vi "Draw Robot.vi"(7 "Gyro":dbl, 10 "XY":cluster{"X":dbl, "Y":dbl}) -> (2 "Graph 2":cluster{cluster{"X":dbl, "Y":dbl}[]}[](graph))   [LabVIEW 2018]
panel:
  in  "Robot Lenght":dbl
  in  "Robot Width":dbl
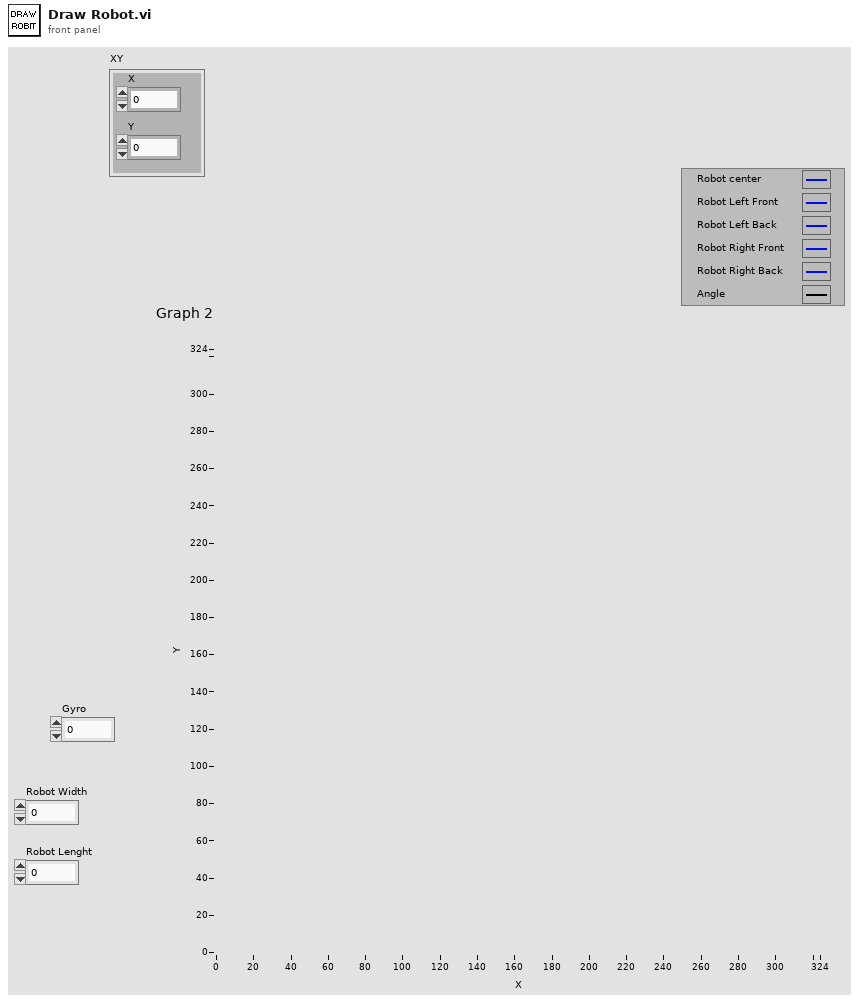
[diagram p1: front panel]
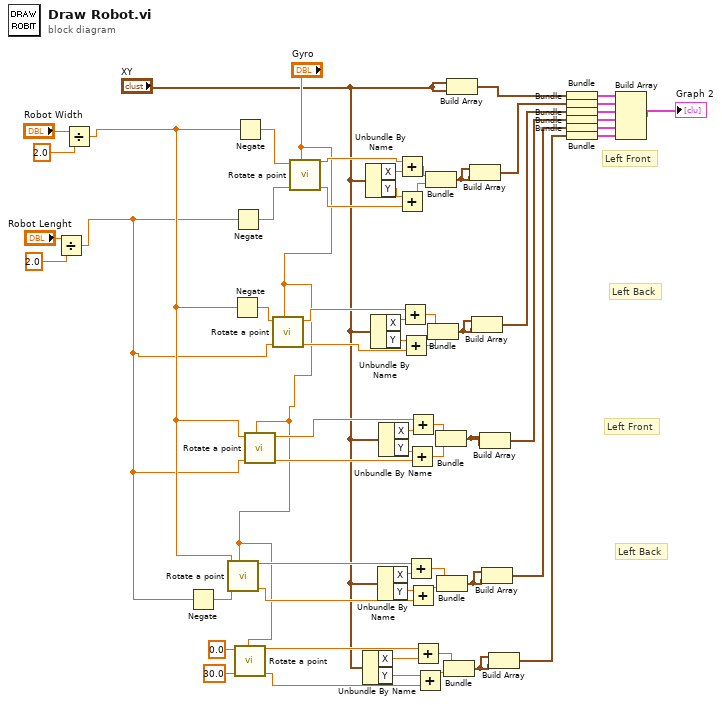
[diagram p0: block diagram]
diagram:
  # "Left Back"
  # "Left Front"
  # "Left Back"
  # "Left Front"
  n1 = Divide(x="Robot Lenght", y=2.0) -> (x/y=w42:dbl)
  n2 = Divide(x="Robot Width", y=2.0) -> (x/y=w43:dbl)
  n3 = Negate(x=w42) -> (-x=w47:dbl)
  n4 = call "Rotate a point.vi"("Gyro"="Gyro", "Y"=w47, "X"=w43) -> ("Y'"=w18:dbl, "X'"=w19:dbl)  [unwired: 7 in]
  n5 = Negate(x=w43) -> (-x=w44:dbl)
  n6 = Negate(x=w42) -> (-x=w45:dbl)
  n7 = Negate(x=w43) -> (-x=w46:dbl)
  n8 = call "Rotate a point.vi"("Gyro"="Gyro", "Y"=30.0, "X"=0.0) -> ("Y'"=w13:dbl, "X'"=w12:dbl)  [unwired: 7 in]
  n9 = call "Rotate a point.vi"("Gyro"="Gyro", "Y"=w42, "X"=w43) -> ("Y'"=w20:dbl, "X'"=w21:dbl)  [unwired: 7 in]
  n10 = call "Rotate a point.vi"("Gyro"="Gyro", "Y"=w42, "X"=w44) -> ("Y'"=w30:dbl, "X'"=w31:dbl)  [unwired: 7 in]
  n11 = call "Rotate a point.vi"("Gyro"="Gyro", "Y"=w45, "X"=w46) -> ("Y'"=w36:dbl, "X'"=w37:dbl)  [unwired: 7 in]
  n12 = Unbundle By Name("XY") -> ("X"=w6:dbl, "Y"=w5:dbl)
  n13 = Unbundle By Name("XY") -> ("X"=w41:dbl, "Y"=w40:dbl)
  n14 = Unbundle By Name("XY") -> ("X"=w34:dbl, "Y"=w33:dbl)
  n15 = Unbundle By Name("XY") -> ("X"=w24:dbl, "Y"=w22:dbl)
  n16 = Unbundle By Name("XY") -> ("X"=w29:dbl, "Y"=w26:dbl)
  n17 = Add(x=w37, y=w41) -> (x+y=w38:dbl)
  n18 = Add(x=w40, y=w36) -> (x+y=w39:dbl)
  n19 = Add(x=w31, y=w34) -> (x+y=w35:dbl)
  n20 = Add(x=w33, y=w30) -> (x+y=w32:dbl)
  n21 = Add(x=w19, y=w24) -> (x+y=w25:dbl)
  n22 = Add(x=w26, y=w20) -> (x+y=w28:dbl)
  n23 = Add(x=w21, y=w29) -> (x+y=w27:dbl)
  n24 = Add(x=w22, y=w18) -> (x+y=w23:dbl)
  n25 = Add(x=w12, y=w6) -> (x+y=w10:dbl)
  n26 = Add(x=w5, y=w13) -> (x+y=w11:dbl)
  n27 = Bundle(w38, w39) -> (w59:cluster{dbl, dbl})  [unwired: 1 in]
  n28 = Bundle(w35, w32) -> (w58:cluster{dbl, dbl})  [unwired: 1 in]
  n29 = Bundle(w27, w28) -> (w55:cluster{dbl, dbl})  [unwired: 1 in]
  n30 = Bundle(w25, w23) -> (w56:cluster{dbl, dbl})  [unwired: 1 in]
  n31 = Bundle(w10, w11) -> (w9:cluster{dbl, dbl})  [unwired: 1 in]
  n32 = Build Array("XY", "XY") -> (w61:cluster{"X":dbl, "Y":dbl}[])
  n33 = Build Array(w59, w59) -> (w60:cluster{dbl, dbl}[])
  n34 = Build Array(w58, w58) -> (w57:cluster{dbl, dbl}[])
  n35 = Build Array(w55, w55) -> (w54:cluster{dbl, dbl}[])
  n36 = Build Array(w56, w56) -> (w53:cluster{dbl, dbl}[])
  n37 = Build Array(w9, w9) -> (w7:cluster{dbl, dbl}[])
  n38 = Bundle(w61) -> (w62:cluster{cluster{"X":dbl, "Y":dbl}[]})  [unwired: 1 in]
  n39 = Bundle(w60) -> (w17:cluster{cluster{dbl, dbl}[]})  [unwired: 1 in]
  n40 = Bundle(w57) -> (w16:cluster{cluster{dbl, dbl}[]})  [unwired: 1 in]
  n41 = Bundle(w54) -> (w15:cluster{cluster{dbl, dbl}[]})  [unwired: 1 in]
  n42 = Bundle(w53) -> (w14:cluster{cluster{dbl, dbl}[]})  [unwired: 1 in]
  n43 = Bundle(w7) -> (w8:cluster{cluster{dbl, dbl}[]})  [unwired: 1 in]
  n44 = Build Array(w62, w17, w16, w15, w14, w8) -> (→"Graph 2":cluster{cluster{"X":dbl, "Y":dbl}[]}[])
